vi "Test Oxford Merc PS.vi"() -> ()   [LabVIEW 2015]
uses:
  PulseEcho/Mercury_IPS/Mercury iXX.lvlib
  PulseEcho/Mercury_IPS/Public/Libraries/System/Open/Open System.vi
  PulseEcho/Mercury_IPS/Public/Libraries/System.lvlib
  PulseEcho/Mercury_IPS/Public/Libraries/Magnet/Open/Open Magnet Device.vi
  PulseEcho/Mercury_IPS/Public/Libraries/Magnet.lvlib
  PulseEcho/Mercury_IPS/Public/Libraries/Magnet/Configuration/Read/Current to Field Factor (Read).vi
  PulseEcho/Mercury_IPS/Public/Libraries/Magnet/Signals/Read/Current (Read).vi
panel:
  out "Response 2":string
  out "Response":string
  in  "VISA resource name":refnum<visa-resource-name>="tcpip::192.168.1.28::7020::socket"
  in  "IP Address":string="192.168.1.28"
  out "AtoB":dbl caption="Current Field Factor (A/T)" format="%#.1f"
  out "Current":dbl
  out "Magnetic Field (T)":dbl
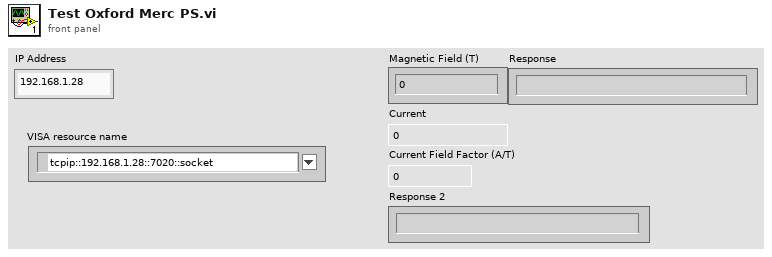
[diagram p1: front panel]
types:
  T1 = typedef "Mercury iXX.lvlib/Mercury Reference.ctl" = cluster{"Comms":refnum<visa-resource-name>, "Device ID":string[], "Comms Layer":T2, "Command":string, "Query reference":T3}
  T2 = typedef "Mercury iXX.lvlib/Comms Transport Layer.ctl" = enum16{"Ethernet TCP/IP", "USB", "ISOBus - RS-232", "GPIB"}
  T3 = typedef "Mercury iXX.lvlib/Query Dynamic Reference.ctl" = refnum<vi>
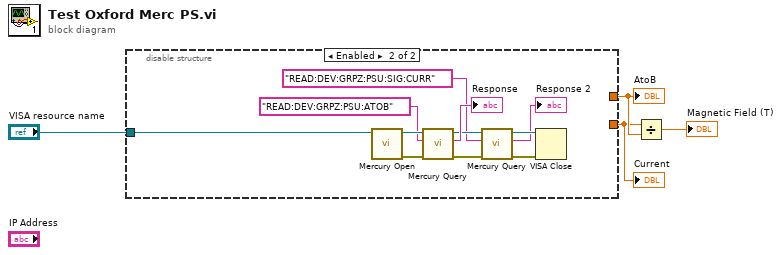
[diagram p0: block diagram]
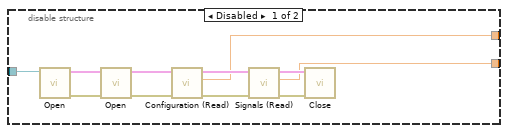
[diagram p2: hidden frame]
diagram:
  n1 = disable-structure shown="Enabled" {
    disable-tunnel: [w7 _] -> w4
    disable-tunnel: [w6 _] -> w3
    disable-tunnel: "VISA resource name" -> [w5 w26]
    frame Disabled {
      n2 = call-poly "Open.vi"("VISA resource name"=w5) -> ("error out"=w9:errorcluster, "Mercury Reference Out"=w8:T1)  [unwired: 6 in, 3 out]
      n3 = call-poly "Open.vi"("error in (no error)"=w9, "Mercury Reference In"=w8) -> ("error out"=w10:errorcluster, "Mercury Reference Out"=w12:T1)  [unwired: 1 in, 7 out]
      n4 = call-poly "Configuration (Read).vi"("error in"=w10, "Mercury Reference In"=w12) -> ("error out"=w11:errorcluster, "AtoB"=w7:dbl, "Mercury Reference Out"=w13:T1)  [unwired: 1 in, 6 out]
      n5 = call-poly "Signals (Read).vi"("error in"=w11, "Mercury Reference In"=w13) -> ("error out"=w15:errorcluster, "Current"=w6:dbl, "Mercury Reference Out"=w14:T1)  [unwired: 1 in, 6 out]
      n6 = call "Close.vi"("error in (no error)"=w15, "Mercury Reference"=w14) -> ()  [unwired: 10 out]
    }
    frame Enabled {
      n7 = call "Mercury Open.vi"("VISA resource name"=w26) -> ("Error Out"=w24:errorcluster, "VISA resource name out"=w25:refnum<visa-resource-name>)  [unwired: 9 in]
      n8 = call "Mercury Query.vi"("Error In"=w24, "Command"="READ:DEV:GRPZ:PSU:ATOB", "VISA resource name"=w25) -> ("Error Out"=w21:errorcluster, "Response"=→"Response":string, "VISA resource name out"=w20:refnum<visa-resource-name>)  [unwired: 6 in]
      n9 = call "Mercury Query.vi"("Error In"=w21, "Command"="READ:DEV:GRPZ:PSU:SIG:CURR", "VISA resource name"=w20) -> ("Error Out"=w17:errorcluster, "Response"=→"Response 2":string, "VISA resource name out"=w18:refnum<visa-resource-name>)  [unwired: 6 in]
      n10 = VISA Close(VISA resource name=w18, error in (no error)=w17) -> ()  [unwired: 1 out]
    }
  }
  "Current" <- w3
  "AtoB" <- w4
  n11 = Divide(x=w3, y=w4) -> (x/y=→"Magnetic Field (T)":dbl)
